vi "ui.vi"() -> ()   [LabVIEW 2018]
uses:
  control/clusterPlatformProfile.ctl
  control/clusterPlatformProfileTheta.ctl
  control/clusterPosition.ctl
  control/clusterPeriod.ctl
  control/clusterSensorState.ctl
  control/clusterPlatformState.ctl
  control/clusterTotalState.ctl
  control/enumTcpCommand.ctl
  <vilib>/Utility/miscctls.llb/LVRectTypeDef.ctl
  control/clusterCustomString.ctl
  <vilib>/Utility/miscctls.llb/LVBoundsTypeDef.ctl
  <vilib>/Utility/miscctls.llb/LVPositionTypeDef.ctl
  control/enumSensorType.ctl
  <vilib>/Utility/miscctls.llb/LVPointTypeDef.ctl
  control/enumFgvFunction.ctl
  <vilib>/Utility/sysdir.llb/System Directory Type.ctl
panel:
  out "Total State":T1={"Sensor State"={"Front"=0.0, "Rear"=0.0, "Right(F)"=0.0, "Righ(R)"=0.0}, "Position State"={"X"=1.0, "Y"=2.0, "Theta"=3.0}, "Platform State"={"Mode"=0, "State"=0}} {"Platform State"."Mode" format="%.0x"; "Platform State"."State" format="%.0x"}
  in  "sensor":T5
  in  "File Name":string
  in  "Save":bool
  in  "Init Platform":bool
  in  "AGV E-Stop":bool
  out "connect?":bool
  out "rx(ms)":u32
  out "tx(ms)":u32
  out "retry":i32
  in  "Tab Control":T6(tab)
  in  "AGV CCW":bool
  in  "AGV CW":bool
  in  "AGV Left":bool
  in  "ARV Right":bool
  in  "AGV Rear":bool
  in  "AGV Front":bool
  in  "Jog Control Velocity Profile Send":bool
  in  "Jog Control Velocity Profile":cluster{"X":T7, "Y":T7, "Theta":T8}={"X"={"Vel/s)"=0.05, "Acc(m/s^2)"=0.1, "Max Vel(m/s)"=0.5}, "Y"={"Vel/s)"=0.05, "Acc(m/s^2)"=0.1, "Max Vel(m/s)"=0.5}, "Theta"={"Vel(deg/s)"=1.0, "Acc(deg/s^2)"=1.0, "Max V(deg/s)"=30.0}}
  out "pos 4":T9(graph)
  out "vel 4":cluster{"value":dbl, "value":dbl, "value":dbl}(graph)
  in  "Position Control Veclocity Profile":cluster{"X":T7, "Y":T7, "Theta":T8}={"X"={"Vel/s)"=0.05, "Acc(m/s^2)"=0.1, "Max Vel(m/s)"=0.5}, "Y"={"Vel/s)"=0.02, "Acc(m/s^2)"=0.02, "Max Vel(m/s)"=0.5}, "Theta"={"Vel(deg/s)"=1.0, "Acc(deg/s^2)"=1.0, "Max V(deg/s)"=30.0}}
  out "vel 3":cluster{"value":dbl, "value":dbl, "value":dbl}(graph)
  in  "Position Control Veclocity Profile Send":bool
  in  "Position Send":bool
  in  "Position":T3
  in  "Pos Control Start":bool
  out "pos 3":T9(graph)
  in  "State Tab Control":enum32{"Request", "Monitor", "Whisper"}(tab)
  out "Get Total(Recv ms)":u32(graph)
  in  "Whisper Data":T10={"Period(ms)"=100}
  in  "Total Data":T10={"Period(ms)"=100}
  in  "Get Total State":bool
  out "Get Total(Recv ms)":u32(graph)
  in  "Get WhisperState":bool
  out "Whisper 1":T11[](array[typedef])
  out "Whisper 2":T11[](array[typedef])
  in  "RecipeLab Tab Control":enum32{"1", "2", "3", "4", "5"}(tab)
  in  "tx string":string
  in  "saving?":bool
  out "tx_packet":string
  out "rx_packet":string
  out "roscore(std out)":string
  out "roscore(std err)":string
  out "roscore(ret)":i32
  out "roscore(err)":errorcluster
  out "rqt(err)":errorcluster
  out "rqt(ret)":i32
  out "rqt(std err)":string
  out "rqt(std out)":string
  in  "roscore":bool
  in  "rqt":bool
  in  "address":string="127.0.0.1"
  in  "port":u16=10100
  in  "tcp rx close?":bool
  in  "send":bool
  out "tx_packet ts":timestamp format="%<%H:%M:%S%3u>T"
  out "rx_packet ts":timestamp format="%<%H:%M:%S%3u>T"
  out "STREAM":timestamp format="%<%H:%M:%S%3u>T"
  out "STREAM Command":T12
  out "ONE":timestamp format="%<%H:%M:%S%3u>T"
  out "ONE Command":T12
  out "RES ts":timestamp format="%<%H:%M:%S%3u>T"
  out "RES Command":T12
  out "ACK Command":T12
  out "ACK ts":timestamp format="%<%H:%M:%S%3u>T"
  in  "Maximize":bool
  out "stop":bool
  in  "AGV Stop(Jog)":bool caption="AGV Stop"
  in  "AGV Stop(Position Control)":bool caption="AGV Stop"
  in  "Command":T12=enum."Set Control Mode"
  in  "Set Control Mode":bool
  in  "Normal Stop(E-Stop)":bool
  in  "Set Jog Control Mode":bool
  in  "Set Position Control Mode":bool
  in  "Position Data":T10={"Period(ms)"=100}
  in  "Sensor Data":T10={"Period(ms)"=100}
  in  "Platform Data":T10={"Period(ms)"=100}
  out "Get Sensor(Recv ms)":u32(graph)
  out "Get Platform(Recv ms)":u32(graph)
  out "Get Position(Recv ms)":u32(graph)
  in  "Get Position State":bool
  in  "Get Sensor State":bool
  in  "Get Platform State":bool
  out "Sensor State":T2
  out "Platform State":T4
  out "Position State":T3={"X"=1.0, "Y"=2.0, "Theta"=3.0}
  in  "Front Panel Window Bounds":T13={"Left"=0, "Top"=27, "Right"=1024, "Bottom"=768}
  out "Position 2":T14
  out "Bounds":T15
  out "Array":cluster{"height":i16, "width":i16}[](array[cluster])
  out "Front Panel Window:Panel Bounds":T13
  out "Front Panel Window:Window Bounds":T13
  # "\"-- mode --\n0xA0: 조그(Jog)\n0xA1: 위치(Pos)\n0xAF: 초기화(Init)\n0xAE: 대기(Ready)\n-- state --\n0xB0: 대기(Ready)\n0xB1: 동작(Run)\""
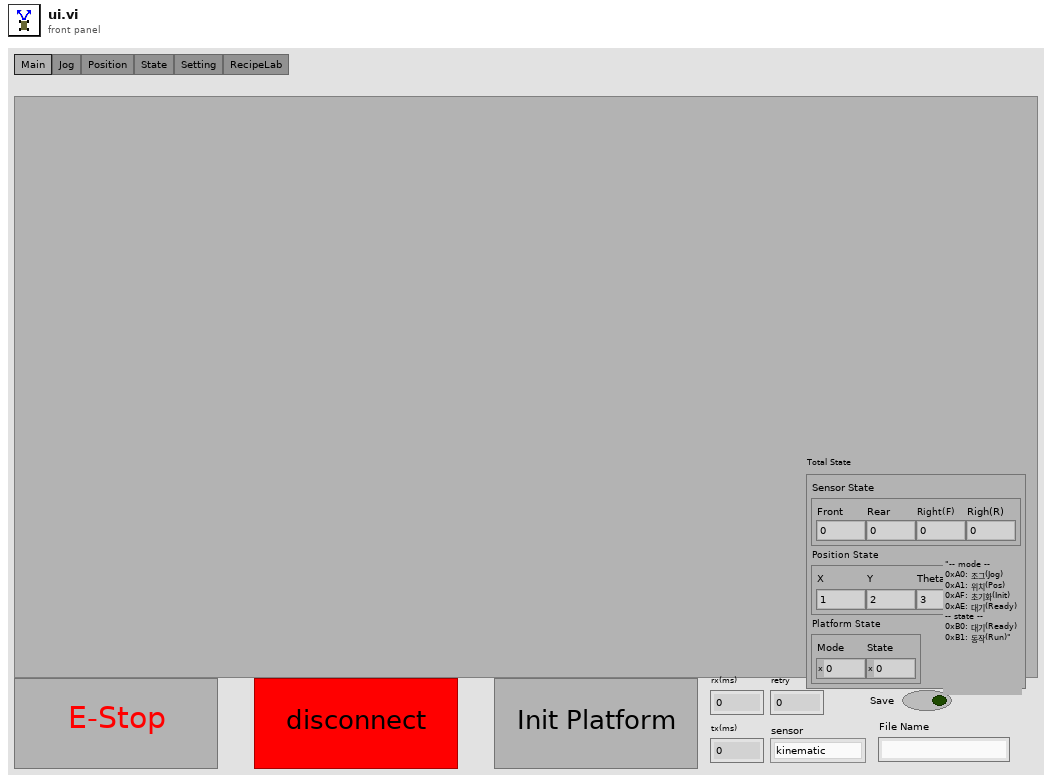
[diagram p1: front panel]
types:
  T1 = typedef "clusterTotalState.ctl" = cluster{"Sensor State":T2, "Position State":T3, "Platform State":T4}
  T2 = typedef "clusterSensorState.ctl" = cluster{"Front":dbl, "Rear":dbl, "Right(F)":dbl, "Righ(R)":dbl}
  T3 = typedef "clusterPosition.ctl" = cluster{"X":dbl, "Y":dbl, "Theta":dbl}
  T4 = typedef "clusterPlatformState.ctl" = cluster{"Mode":i32, "State":i32}
  T5 = typedef "enumSensorType.ctl" = enum16{"kinematic", "1d lidar", "fusion"}
  T6 = enum32{"Main", "Jog", "Position", "State", "Setting", "RecipeLab"}
  T7 = typedef "clusterPlatformProfile.ctl" = cluster{"Vel/s)":dbl, "Acc(m/s^2)":dbl, "Max Vel(m/s)":dbl}
  T8 = typedef "clusterPlatformProfileTheta.ctl" = cluster{"Vel(deg/s)":dbl, "Acc(deg/s^2)":dbl, "Max V(deg/s)":dbl}
  T9 = cluster{"value":dbl, "value":dbl, "value":dbl, "value":dbl, "value":dbl, "value":dbl}
  T10 = typedef "clusterPeriod.ctl" = cluster{"Period(ms)":i32}
  T11 = typedef "clusterCustomString.ctl" = cluster{"subject":string, "value":dbl}
  T12 = typedef "enumTcpCommand.ctl" = enum16{"None", "Stop", "E-Stop", "Set Position Control Mode", "Set Jog Control Mode", "Set Control Mode", "Set Jog Control Profile Parameter", "Set Position Control Profile Parameter", "Set Jog State", "Set Position", "Start Position Control", "Get Total State", "Get Platform State", "Get Sensor State", "Get Position State", "Init Platform", "Get Whisper State", "Set Sensor"}
  T13 = typedef "LVRectTypeDef.ctl" = cluster{"Left":i16, "Top":i16, "Right":i16, "Bottom":i16}
  T14 = typedef "LVPositionTypeDef.ctl" = cluster{"Left":i32, "Top":i32}
  T15 = typedef "LVBoundsTypeDef.ctl" = cluster{"Width":u32, "Height":u32}
  T16 = enum32{"invalid app kind", "Development System", "Run Time System", "Student Edition", "Embedded LabVIEW", "Evaluation", "Custom"}
  T17 = typedef "LVPointTypeDef.ctl" = cluster{"Horizontal":i16, "Vertical":i16}
  T18 = typedef "enumFgvFunction.ctl" = enum16{"Open", "Read", "Check", "Write", "Close"}
  T19 = cluster{"subject":u64, "subject":i64, "val_dbl":dbl}[]
  T20 = typedef "System Directory Type.ctl" = i32
  T21 = cluster{"[0]":u32, "[1]":u32, "[2]":u32, "[3]":u32, "[4]":u32, "[5]":u32}
  T22 = enum16{"Always On", "Always Off", "Off While Running"}
  T23 = enum16{"Standard", "Buffered", "CRLF", "Immediate"}
  T24 = cluster{cluster{dbl, dbl, dbl, dbl}, cluster{dbl, dbl, dbl}, cluster{i32, i32}}
  T25 = cluster{"double[0]":dbl, "double[1]":dbl, "double[2]":dbl, "double[3]":dbl}
  T26 = cluster{"double[0]":dbl, "double[1]":dbl, "double[2]":dbl}
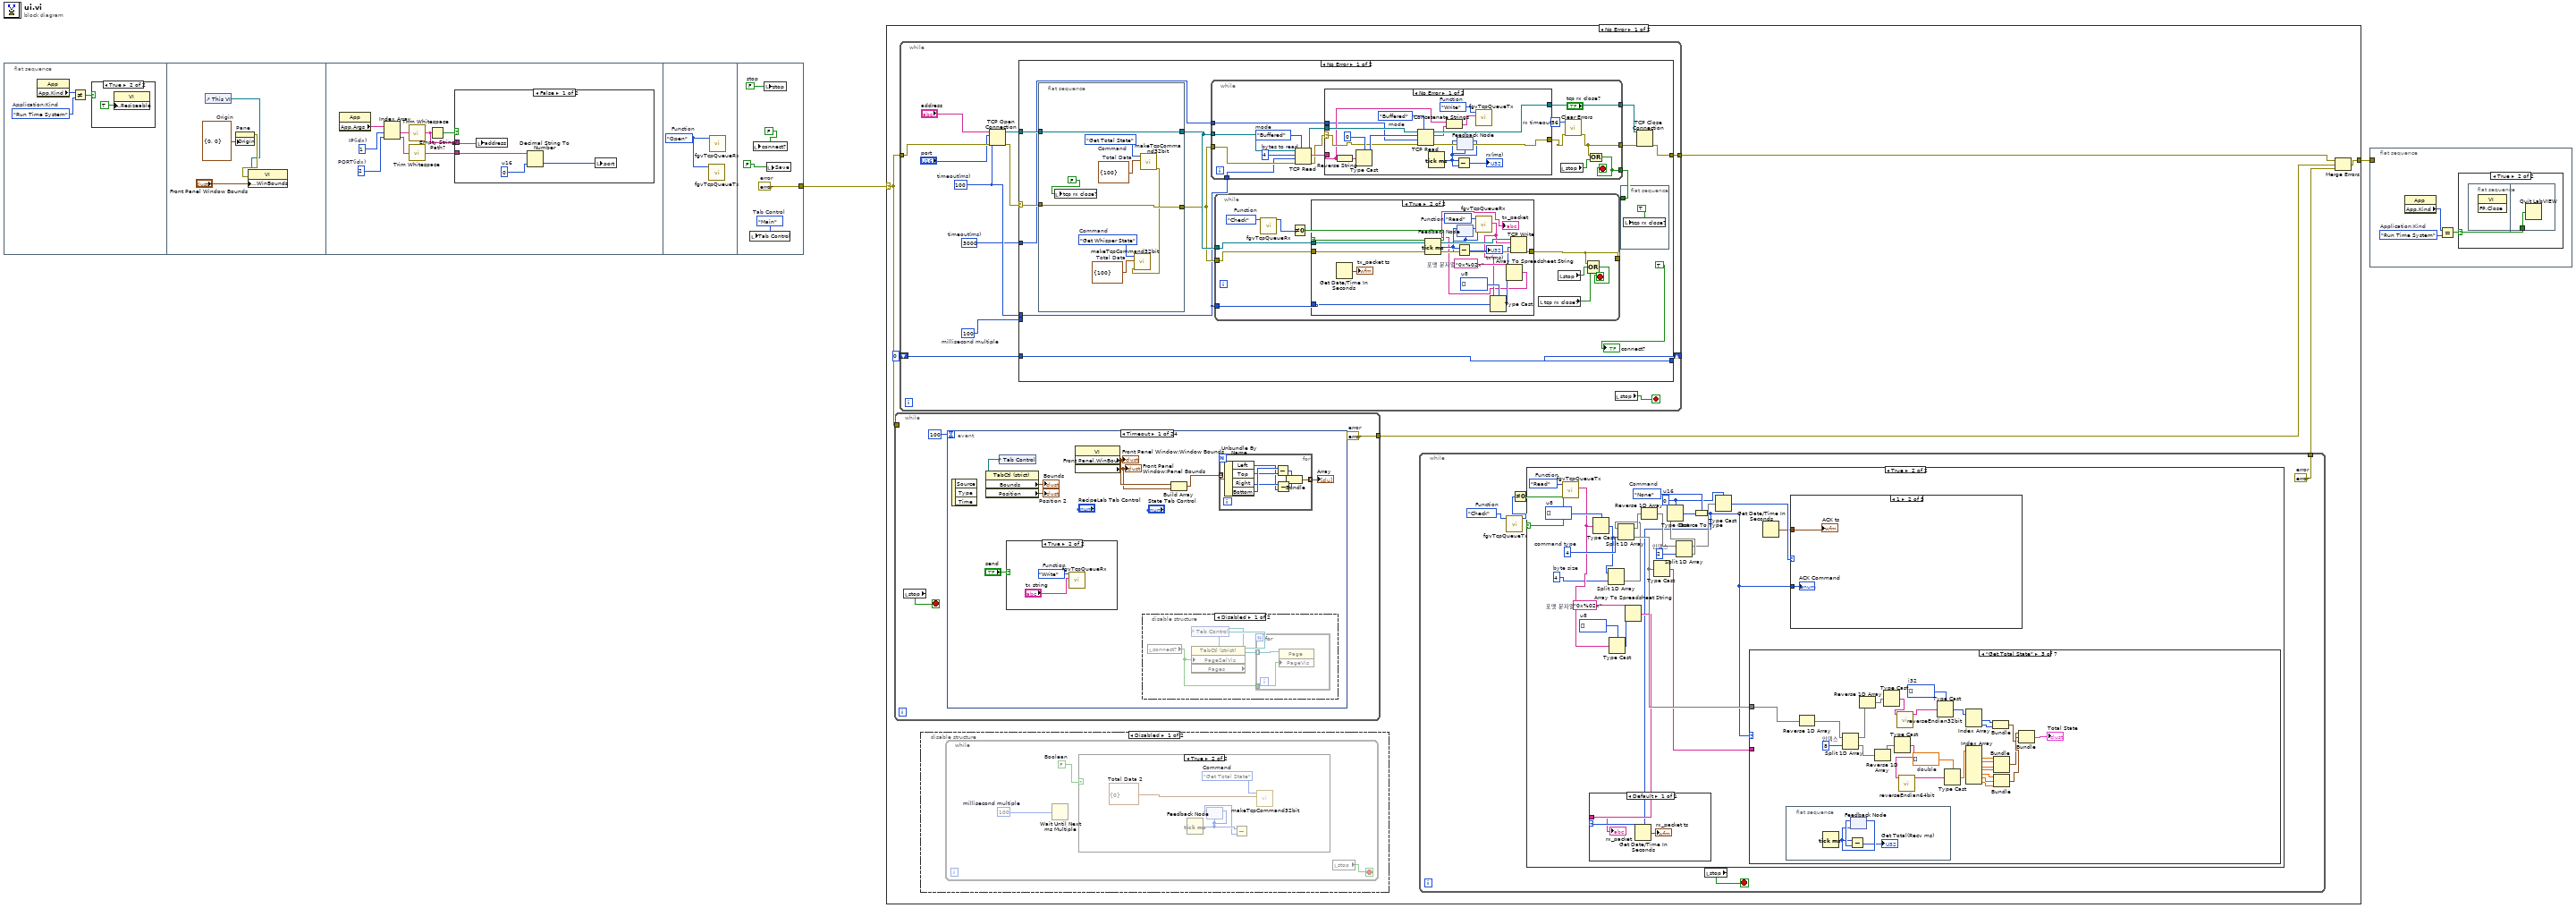
[diagram p0: block diagram]
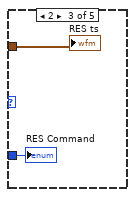
[diagram p6: hidden frame]
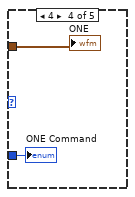
[diagram p7: hidden frame]
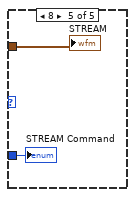
[diagram p8: hidden frame]
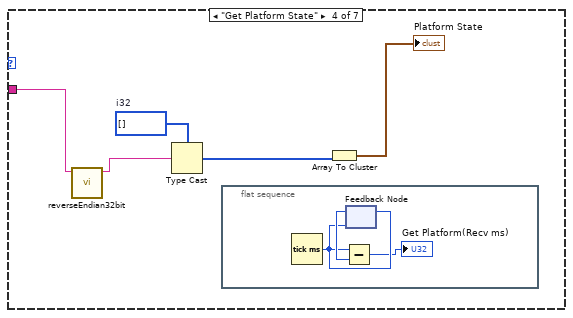
[diagram p11: hidden frame]
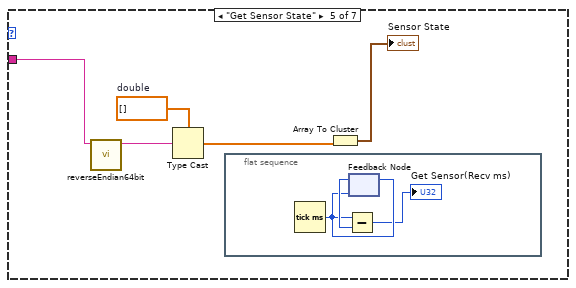
[diagram p12: hidden frame]
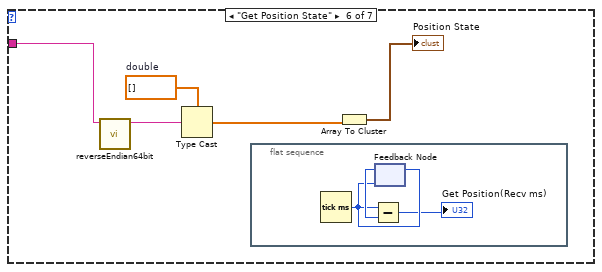
[diagram p13: hidden frame]
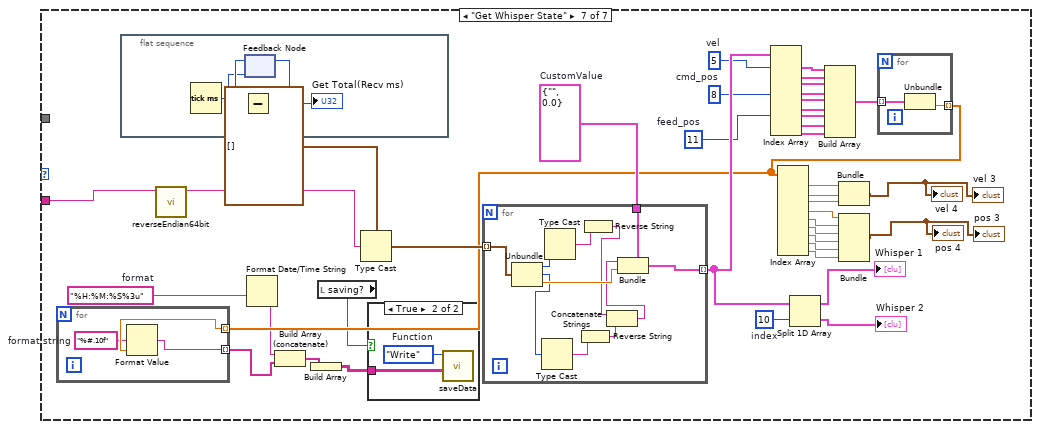
[diagram p14: hidden frame]
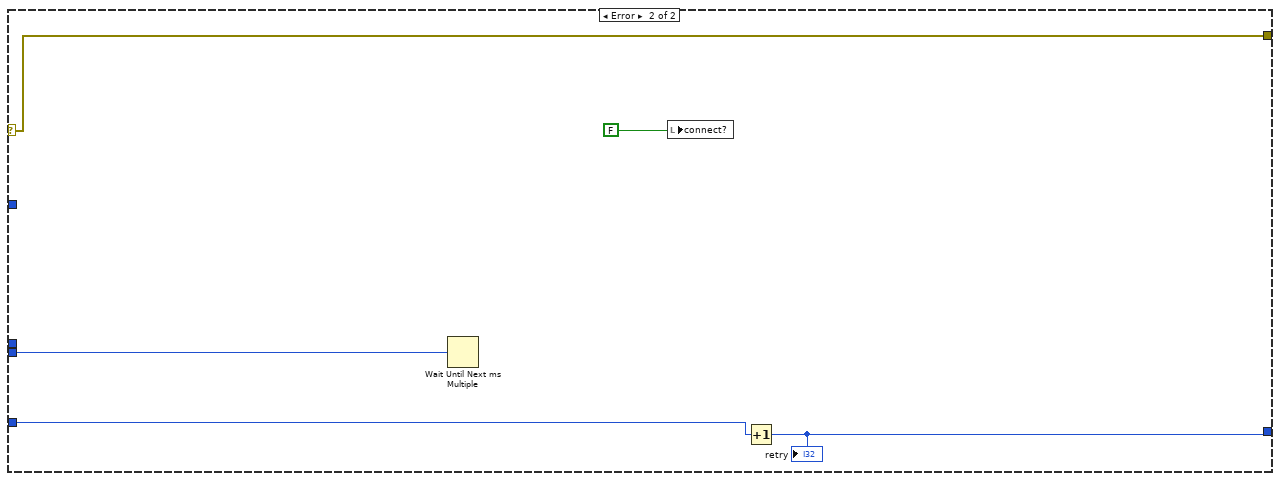
[diagram p18: hidden frame]
diagram:
  n1 = flat-sequence {
    tunnel: [w27] -> w1
    frame #0 {
      w3 = T16."Run Time System"  # Application:Kind
      n2 = property class="App"() -> ("App.Kind"=w4:T16)  [unwired: 2 in, 2 out]
      n3 = Not Equal?(x=w4, y=w3) -> (x != y?=w5:bool)
      n4 = case shown="True" w5 {
        frame False {
        }
        frame True {
          n5 = property class="VI"("Front Panel.Resizeable"=TRUE) -> ()  [unwired: 2 in, 2 out]
        }
      }
    }
    frame #1 {
      w10 = T17 {"Horizontal"=0, "Vertical"=0}  # Origin
      n6 = control-ref of="This VI"() -> (w8:refnum<vi>)
      n7 = property on="Pane" class="Pane"("Origin"=w10) -> (error out=w9:errorcluster)  [unwired: 2 in, 1 out]
      n8 = property on="Property Node" class="VI"(reference=w8, error in=w9, "Front Panel.WinBounds"="Front Panel Window Bounds") -> ()  [unwired: 2 out]
    }
    frame #2 {
      w16 = 2  # PORT(idx)
      w17 = 1  # IP(idx)
      n9 = property class="App"() -> ("App.Args"=w18:string[])  [unwired: 2 in, 2 out]
      n10 = Index Array(array=w18, index #1=w17, index #2=w16) -> (element #1=w15:string, element #2=w14:string)
      n11 = call <vilib>:"Trim Whitespace.vi"("string"=w15) -> ("trimmed string"=w13:string)  [unwired: 1 in]
      n12 = call <vilib>:"Trim Whitespace.vi"("string"=w14) -> ("trimmed string"=w12:string)  [unwired: 1 in]
      n13 = Empty String/Path?(string/path=w13) -> (empty?=w11:bool)
      n14 = case shown="False" w11 {
        tunnel: w13 -> [w22 _]
        tunnel: w12 -> [w21 _]
        frame False {
          w19 = u16 0  # u16
          n15 = local write "address"(w22) -> ()
          n16 = Decimal String To Number(string=w21, default (0L)=w19) -> (number=w20:u16)  [unwired: 1 in, 1 out]
          n17 = local write "port"(w20) -> ()
        }
        frame True {
        }
      }
    }
    frame #3 {
      w23 = enumFgvFunction."Open"  # Function
      n18 = call "fgvTcpQueueTx.vi"("Function"=w23) -> ()  [unwired: 8 in, 3 out]
      n19 = call "fgvTcpQueueRx.vi"("Function"=w23) -> ()  [unwired: 8 in, 3 out]
    }
    frame #4 {
      w24 = T6."Main"  # Tab Control
      w27 = errorcluster {"status"=FALSE, "code"=0, "source"=""}  # error
      w28 = FALSE  # stop
      n20 = local write "Tab Control"(w24) -> ()
      n21 = local write "connect?"(FALSE) -> ()
      n22 = local write "stop"(w28) -> ()
      n23 = local write "Save"(FALSE) -> ()
    }
  }
  n24 = case shown="No Error" w1 {
    selector: w1 -> [w32 w422]
    tunnel: [w33 w422] -> w2
    frame No Error {
      n25 = while {
        tunnel: w32 -> [_]
        tunnel: [w293] -> w34
        stop <- w295 stop-if-true
        w293 = errorcluster {"status"=FALSE, "code"=0, "source"=""}  # error
        n26 = local read "stop"() -> (w295:bool)
        n27 = event shown="[0] Timeout" {
          selector: _ -> [_ _ _ _ _ _ _ _ _ _ _ _ _ _ _ _ _ _ _ _ _ _ _ _]
          dyn-events: _ -> [_ _ _ _ _ _ _ _ _ _ _ _ _ _ _ _ _ _ _ _ _ _ _ _]
          timeout: 100 -> [_ _ _ _ _ _ _ _ _ _ _ _ _ _ _ _ _ _ _ _ _ _ _ _]
          event Timeout {
            n28 = event-data() -> ()  [unwired: 1 in, 3 out]
            n29 = control-ref of="Tab Control"() -> (w299:refnum<vi>)
            n30 = property on="Property Node" class="TabCtl (strict)"(reference=w299) -> ("Bounds"=→"Bounds":T15, "Position"=→"Position 2":T14)  [unwired: 1 in, 2 out]
            n31 = case shown="True" "send" {
              frame False {
              }
              frame True {
                w305 = enumFgvFunction."Write"  # Function
                n32 = call "fgvTcpQueueRx.vi"("Write"="tx string", "Function"=w305) -> ()  [unwired: 7 in, 3 out]
              }
            }
            n33 = property on="Property Node" class="VI"() -> ("Front Panel.WinBounds"=w303:T13, "Front Panel.PanelBounds"=w302:T13)  [unwired: 2 in, 2 out]
            "Front Panel Window:Window Bounds" <- w303
            "Front Panel Window:Panel Bounds" <- w302
            n34 = disable-structure shown="Disabled" {
              frame Disabled {
                n35 = local read "connect?"() -> (w306:bool)
                n36 = control-ref of="Tab Control"() -> (w308:refnum<vi>)
                n37 = property class="TabCtl (strict)"(reference=w308, "PageSelVis"=w306) -> ("Pages"=w307:refnum<vi>[])  [unwired: 1 in, 2 out]
                n38 = for {
                  tunnel: w307 -> [w310] mode=indexing
                  tunnel: w306 -> [w309]
                  n39 = property class="Page"(reference=w310, "PageVis"=w309) -> ()  [unwired: 1 in, 2 out]
                }
              }
              frame Enabled {
              }
            }
            n40 = Build Array(w303, w302) -> (w301:T13[])
            n41 = for {
              tunnel: w301 -> [w318] mode=indexing
              tunnel: [w311] -> w300 mode=indexing
              n42 = Unbundle By Name(w318) -> ("Left"=w314:i16, "Top"=w316:i16, "Right"=w315:i16, "Bottom"=w317:i16)
              n43 = Subtract(x=w317, y=w316) -> (x-y=w313:i16)
              n44 = Subtract(x=w315, y=w314) -> (x-y=w312:i16)
              n45 = Bundle(w313, w312) -> (w311:cluster{i16, i16})  [unwired: 1 in]
            }
            "Array" <- w300
          }
          event Value Change {
            w321 = enumTcpCommand."Set Sensor"  # Command
            n46 = event-data() -> ()  [unwired: 1 in, 6 out]
            n47 = To Unsigned Long Integer(number="sensor") -> (unsigned 32bit integer=w319:u32)
            n48 = call "makeTcpCommand32bit.vi"("Variant"=w319, "Command"=w321) -> ()  [unwired: 7 in, 3 out]
          }
          event "Tab Control": Value Change {
            n49 = event-data() -> ("OldVal"=w324:T6, "NewVal"=w322:T6)  [unwired: 1 in, 4 out]
            n50 = Not Equal?(x=w324, y=w322) -> (x != y?=w323:bool)
            n51 = case shown="True" w323 {
              tunnel: w322 -> [_ w325]
              frame False {
              }
              frame True {
                n52 = case shown="\"Jog\"" w325 {
                  frame Default {
                  }
                  frame "Jog" {
                    w327 = enumTcpCommand."Set Jog Control Profile Parameter"  # Command
                    w329 = enumTcpCommand."Set Jog Control Mode"  # Command
                    n53 = call "makeTcpCommand32bit.vi"("Command"=w329) -> ("error out"=w326:errorcluster)  [unwired: 8 in, 2 out]
                    n54 = local read "Jog Control Velocity Profile"() -> (w328:cluster{"X":T7, "Y":T7, "Theta":T8})
                    n55 = call "makeTcpCommand64bit.vi"("error in"=w326, "Variant"=w328, "Command"=w327) -> ()  [unwired: 6 in, 3 out]
                  }
                  frame "Position" {
                    w331 = enumTcpCommand."Set Position Control Profile Parameter"  # Command
                    w333 = enumTcpCommand."Set Position Control Mode"  # Command
                    n56 = call "makeTcpCommand32bit.vi"("Command"=w333) -> ("error out"=w330:errorcluster)  [unwired: 8 in, 2 out]
                    n57 = local read "Position Control Veclocity Profile"() -> (w332:cluster{"X":T7, "Y":T7, "Theta":T8})
                    n58 = call "makeTcpCommand64bit.vi"("error in"=w330, "Variant"=w332, "Command"=w331) -> ()  [unwired: 6 in, 3 out]
                  }
                }
              }
            }
          }
          event "Save": Value Change {
            n59 = event-data() -> ("NewVal"=w335:bool)  [unwired: 1 in, 5 out]
            n60 = case shown="False" w335 {
              tunnel: [FALSE TRUE] -> w334
              frame False {
                w337 = enumFgvFunction."Close"  # Function
                n61 = call "saveData.vi"("Function"=w337) -> ()  [unwired: 8 in, 3 out]
              }
              frame True {
                w338 = "_"  # string
                w343 = string[][] [["timestamp", "vel.x", "vel.y", "vel.rx", "cmdx", "cmdy", "cmdz", "feedx", "feedy", "feedz"]]  # header
                w346 = T20 0 items=["User Home"=0, "User Desktop"=1, "User Documents"=2, "User Application Data"=3, "User Preferences"=4, "User Temporary"=5, "Public Documents"=6, "Public Application Data"=7, "Public Preferences"=8, "Public Cache"=13, "System Core Libraries"=9, "System Installed Libraries"=10, "Application Files"=11, "Boot Volume Root"=12]  # system directory type
                w348 = enumFgvFunction."Open"  # Function
                n62 = call <vilib>:"Get System Directory.vi"("system directory type"=w346) -> ("system directory"=w345:path)  [unwired: 10 in]
                n63 = control-ref of="This VI"() -> (w342:refnum<vi>)
                n64 = Format Date/Time String(time format string (%c)="%Y%m%d_%H%M%S") -> (date/time string=w341:string)  [unwired: 2 in]
                n65 = Concatenate Strings(w341, w338, "File Name") -> (w339:string)
                n66 = call "saveData.vi"("file name"=w339, "이미지 저장 VI"=w342, "file path 경로"=w345, "header"=w343, "Function"=w348) -> ()  [unwired: 4 in, 3 out]
              }
            }
            n67 = local write "saving?"(w334) -> ()
          }
          event "roscore": Value Change {
            n68 = event-data() -> ()  [unwired: 1 in, 6 out]
            n69 = call <vilib>:"System Exec.vi"("wait until completion? (T)"=FALSE, "command line"="roscore") -> ("error out"=→"roscore(err)":errorcluster, "return code"=→"roscore(ret)":i32, "standard error"=→"roscore(std err)":string, "standard output"=→"roscore(std out)":string)  [unwired: 6 in]
          }
          event "Position Control Veclocity Profile Send": Value Change {
            w356 = enumTcpCommand."Set Position Control Profile Parameter"  # Command
            n70 = event-data() -> ()  [unwired: 1 in, 6 out]
            n71 = call "makeTcpCommand64bit.vi"("Variant"="Position Control Veclocity Profile", "Command"=w356) -> ()  [unwired: 7 in, 3 out]
          }
          event "Jog Control Velocity Profile Send": Value Change {
            w358 = enumTcpCommand."Set Jog Control Profile Parameter"  # Command
            n72 = event-data() -> ()  [unwired: 1 in, 6 out]
            n73 = call "makeTcpCommand64bit.vi"("Variant"="Jog Control Velocity Profile", "Command"=w358) -> ()  [unwired: 7 in, 3 out]
          }
          event "AGV Front", "AGV Rear", "ARV Right", "AGV Left", "AGV CW", "AGV CCW": Value Change {
            w364 = enumTcpCommand."Set Jog State"  # Command
            n74 = event-data() -> ()  [unwired: 1 in, 6 out]
            n75 = Build Array("AGV Front", "AGV Rear", "AGV Left", "ARV Right", "AGV CW", "AGV CCW") -> (w365:bool[])
            n76 = Boolean To (0,1)(Boolean=w365) -> (0, 1=w363:i16[])
            n77 = To Unsigned Long Integer(number=w363) -> (unsigned 32bit integer=w360:u32[])
            n78 = Array To Cluster(array=w360) -> (cluster=w359:T21)
            n79 = call "makeTcpCommand32bit.vi"("Variant"=w359, "Command"=w364) -> ()  [unwired: 7 in, 3 out]
          }
          event "Set Jog Control Mode": Value Change {
            w370 = enumTcpCommand."Set Jog Control Mode"  # Command
            n80 = event-data() -> ()  [unwired: 1 in, 6 out]
            n81 = call "makeTcpCommand32bit.vi"("Command"=w370) -> ()  [unwired: 8 in, 3 out]
          }
          event "Set Control Mode": Value Change {
            w374 = enumTcpCommand."Set Control Mode"  # Command
            n82 = event-data() -> ()  [unwired: 1 in, 6 out]
            n83 = To Unsigned Long Integer(number="Command") -> (unsigned 32bit integer=w372:u32)
            n84 = Bundle(w372) -> (w371:cluster{u32})  [unwired: 1 in]
            n85 = call "makeTcpCommand32bit.vi"("Variant"=w371, "Command"=w374) -> ()  [unwired: 7 in, 3 out]
          }
          event "Init Platform": Value Change {
            w375 = enumTcpCommand."Init Platform"  # Command
            n86 = event-data() -> ()  [unwired: 1 in, 6 out]
            n87 = call "makeTcpCommand32bit.vi"("Command"=w375) -> ()  [unwired: 8 in, 3 out]
          }
          event "Set Position Control Mode": Value Change {
            w376 = enumTcpCommand."Set Position Control Mode"  # Command
            n88 = event-data() -> ()  [unwired: 1 in, 6 out]
            n89 = call "makeTcpCommand32bit.vi"("Command"=w376) -> ()  [unwired: 8 in, 3 out]
          }
          event "AGV E-Stop": Value Change {
            w377 = enumTcpCommand."E-Stop"  # Command
            n90 = event-data() -> ()  [unwired: 1 in, 6 out]
            n91 = call "makeTcpCommand32bit.vi"("Command"=w377) -> ()  [unwired: 8 in, 3 out]
          }
          event "Pos Control Start": Value Change {
            w378 = enumTcpCommand."Start Position Control"  # Command
            n92 = event-data() -> ()  [unwired: 1 in, 6 out]
            n93 = call "makeTcpCommand32bit.vi"("Command"=w378) -> ()  [unwired: 8 in, 3 out]
          }
          event "Get Total State": Value Change {
            w380 = enumTcpCommand."Get Total State"  # Command
            n94 = event-data() -> ()  [unwired: 1 in, 6 out]
            n95 = call "makeTcpCommand32bit.vi"("Variant"="Total Data", "Command"=w380) -> ()  [unwired: 7 in, 3 out]
          }
          event "Get Sensor State": Value Change {
            w382 = enumTcpCommand."Get Sensor State"  # Command
            n96 = event-data() -> ()  [unwired: 1 in, 6 out]
            n97 = call "makeTcpCommand32bit.vi"("Variant"="Sensor Data", "Command"=w382) -> ()  [unwired: 7 in, 3 out]
          }
          event "Get Position State": Value Change {
            w384 = enumTcpCommand."Get Position State"  # Command
            n98 = event-data() -> ()  [unwired: 1 in, 6 out]
            n99 = call "makeTcpCommand32bit.vi"("Variant"="Position Data", "Command"=w384) -> ()  [unwired: 7 in, 3 out]
          }
          event "Get Platform State": Value Change {
            w386 = enumTcpCommand."Get Platform State"  # Command
            n100 = event-data() -> ()  [unwired: 1 in, 6 out]
            n101 = call "makeTcpCommand32bit.vi"("Variant"="Platform Data", "Command"=w386) -> ()  [unwired: 7 in, 3 out]
          }
          event "Get WhisperState": Value Change {
            w388 = enumTcpCommand."Get Whisper State"  # Command
            n102 = event-data() -> ()  [unwired: 1 in, 6 out]
            n103 = call "makeTcpCommand32bit.vi"("Variant"="Whisper Data", "Command"=w388) -> ()  [unwired: 7 in, 3 out]
          }
          event "AGV Stop(Jog)", "AGV Stop(Position Control)": Value Change {
            n104 = event-data() -> ("CtlRef"=w391:refnum<vi>, "NewVal"=w389:bool)  [unwired: 1 in, 4 out]
            n105 = property class="Bool (strict)"(reference=w391) -> ("Label.Text"=w390:string)  [unwired: 1 in, 2 out]
            n106 = case shown="\"AGV Stop(Position Control)\"" w390 {
              tunnel: w389 -> [_ w396 w397]
              frame Default {
              }
              frame "AGV Stop(Jog)" {
                n107 = local write "AGV Stop(Position Control)"(w396) -> ()
              }
              frame "AGV Stop(Position Control)" {
                n108 = local write "AGV Stop(Jog)"(w397) -> ()
              }
            }
            n109 = case shown="True" w389 {
              frame False {
              }
              frame True {
                w394 = enumTcpCommand."Stop"  # Command
                n110 = Boolean To (0,1)(Boolean="Normal Stop(E-Stop)") -> (0, 1=w395:i16)
                n111 = To Unsigned Long Integer(number=w395) -> (unsigned 32bit integer=w393:u32)
                n112 = call "makeTcpCommand32bit.vi"("Variant"=w393, "Command"=w394) -> ()  [unwired: 7 in, 3 out]
              }
            }
          }
          event "Maximize": Value Change {
            w398 = T22."Off While Running"  # Horizontal Scrollbar Visibility
            w401 = FALSE  # Tool Bar:Visible
            w402 = FALSE  # Front Panel Window:Show Menu Bar
            w403 = T13 {"Left"=0, "Top"=27, "Right"=1024, "Bottom"=768}  # Front Panel Window:Panel Bounds
            w404 = TRUE  # Front Panel Window:Is Frontmost
            n113 = event-data() -> ()  [unwired: 1 in, 6 out]
            n114 = control-ref of="This VI"() -> (w405:refnum<vi>)
            n115 = property class="VI" props=["Front Panel.IsFrontmost", "Front Panel.PanelBounds", "Front Panel.ShowMenuBar", "TB.Visible", "Clone Name"](reference=w405, "Front Panel.IsFrontmost"=w404, "Front Panel.PanelBounds"=w403, "Front Panel.ShowMenuBar"=w402, "TB.Visible"=w401) -> (error out=w400:errorcluster)  [unwired: 1 in, 2 out]
            n116 = control-ref of="Pane"() -> (w399:refnum<vi>)
            n117 = property class="Pane"(reference=w399, error in=w400, "HorizScrollbarVisibility"=w398, "VertScrollbarVisibility"=w398) -> ()  [unwired: 2 out]
          }
          event "Position Send": Value Change {
            w407 = enumTcpCommand."Set Position"  # Command
            n118 = event-data() -> ()  [unwired: 1 in, 6 out]
            n119 = call "makeTcpCommand64bit.vi"("Variant"="Position", "Command"=w407) -> ()  [unwired: 7 in, 3 out]
          }
          event "rqt": Value Change {
            n120 = event-data() -> ()  [unwired: 1 in, 6 out]
            n121 = call <vilib>:"System Exec.vi"("wait until completion? (T)"=FALSE, "command line"="rqt") -> ("error out"=→"rqt(err)":errorcluster, "return code"=→"rqt(ret)":i32, "standard error"=→"rqt(std err)":string, "standard output"=→"rqt(std out)":string)  [unwired: 6 in]
          }
          event Panel Close? {
            w414 = TRUE  # stop
            n122 = event-data() -> ()  [unwired: 1 in, 4 out]
            n123 = disable-structure shown="Enabled" {
              disable-tunnel: [w416 TRUE] -> w415
              frame Disabled {
                w418 = T16."Run Time System"  # Application:Kind
                n124 = property class="App"() -> ("App.Kind"=w419:T16)  [unwired: 2 in, 2 out]
                n125 = Equal?(x=w419, y=w418) -> (x = y?=w417:bool)
                n126 = Not(x=w417) -> (.not. x?=w416:bool)
              }
              frame Enabled {
              }
            }
            n127 = event-data("Discard?"=w415) -> ()  [unwired: 1 in, 1 out]
            "stop" <- w414
          }
        }
      }
      n128 = while {
        tunnel: w32 -> [w207]
        tunnel: [w206] -> w31
        shift-right: [w201] -> _
        shift-left: 0 -> [w200]
        stop <- w208 stop-if-true
        w197 = 3000  # timeout(ms)
        w199 = u32 100  # millisecond multiple
        w198 = 100  # timeout(ms)
        n129 = TCP Open Connection(address="address", remote port or service name="port", timeout ms (60000)=w198, error in (no error)=w207) -> (connection ID=w203:refnum<k5>, error out=w202:errorcluster)  [unwired: 1 in]
        n130 = case shown="No Error" w202 {
          selector: w202 -> [w212 w292]
          tunnel: [w219 w292] -> w206
          tunnel: w203 -> [w214 _]
          tunnel: [w217 w290] -> w201
          tunnel: w200 -> [w217 w291]
          tunnel: w199 -> [_ w288]
          tunnel: w198 -> [w211 _]
          tunnel: w197 -> [w210 _]
          frame No Error {
            n131 = flat-sequence {
              tunnel: [w229] -> w215
              tunnel: w214 -> [w229]
              tunnel: [w228] -> w213
              tunnel: w212 -> [w228]
              frame #0 {
                w225 = T10 {"Period(ms)"=100}  # Total Data
                w224 = enumTcpCommand."Get Whisper State"  # Command
                w226 = T10 {"Period(ms)"=100}  # Total Data
                w227 = enumTcpCommand."Get Total State"  # Command
                n132 = local write "tcp rx close?"(FALSE) -> ()
                n133 = call "makeTcpCommand32bit.vi"("Variant"=w226, "Command"=w227) -> ("error out"=w223:errorcluster)  [unwired: 7 in, 2 out]
                n134 = call "makeTcpCommand32bit.vi"("error in"=w223, "Variant"=w225, "Command"=w224) -> ()  [unwired: 6 in, 3 out]
              }
            }
            n135 = while {
              tunnel: w213 -> [w269]
              tunnel: [w259] -> w220
              tunnel: w215 -> [w268]
              tunnel: [w262] -> w218
              tunnel: w211 -> [w257]
              tunnel: w210 -> [w256]
              tunnel: [w255] -> w209
              stop <- w255 stop-if-true
              w258 = 56  # rx timeout
              w266 = 4  # bytes to read
              w267 = T23."Buffered"  # mode
              n136 = TCP Read(connection ID=w268, bytes to read=w266, error in (no error)=w269, 7:w267, 9:w257) -> (connection ID out=w264:refnum<k5>, data out=w263:string, error out=w261:errorcluster)
              n137 = case shown="No Error" w261 {
                selector: w261 -> [w277 w287]
                tunnel: w264 -> [w284 w286]
                tunnel: w263 -> [w273 _]
                tunnel: [w280 w286] -> w262
                tunnel: [w279 w287] -> w260
                tunnel: w256 -> [w270 _]
                frame No Error {
                  w278 = enumFgvFunction."Write"  # Function
                  w285 = T23."Buffered"  # mode
                  n138 = Reverse String(1:w273) -> (0:w283:string)
                  n139 = Type Cast(type=0, x=w283) -> (*(type *) &x=w282:i32)
                  n140 = TCP Read(connection ID=w284, bytes to read=w282, error in (no error)=w277, 7:w285, 9:w270) -> (connection ID out=w280:refnum<k5>, data out=w272:string, error out=w279:errorcluster)
                  n141 = Tick Count (ms)() -> (millisecond timer value=w275:u32)
                  n142 = Concatenate Strings(w273, w272) -> (w271:string)
                  n143 = feedback #1(w275) -> (w274:u32)
                  n144 = Subtract(x=w275, y=w274) -> (x-y=→"rx(ms)":u32)
                  n145 = feedback-in #1(w275) -> ()
                  n146 = call "fgvTcpQueueTx.vi"("Write"=w271, "Function"=w278) -> ()  [unwired: 7 in, 3 out]
                }
                frame Error {
                }
              }
              n147 = local read "stop"() -> (w265:bool)
              n148 = call <vilib>:"Clear Errors.vi"("error in (no error)"=w260, "specific error code to clear (0: all)"=w258) -> ("error out"=w259:errorcluster)  [unwired: 4 in, 1 out]
              n149 = Compound Arithmetic op=OR(w259, w265) -> (w255:bool)
            }
            n150 = while {
              tunnel: w213 -> [w231]
              tunnel: [w239] -> _
              tunnel: w215 -> [w233]
              tunnel: w211 -> [w232]
              stop <- w237 stop-if-true
              w236 = enumFgvFunction."Check"  # Function
              n151 = call "fgvTcpQueueRx.vi"("Function"=w236) -> ("Count"=w235:i32)  [unwired: 8 in, 2 out]
              n152 = Not Equal To 0?(x=w235) -> (x != 0?=w234:bool)
              n153 = case shown="True" w234 {
                tunnel: [w240 w254] -> w239
                tunnel: w231 -> [w240 w253]
                tunnel: w233 -> [_ w252]
                tunnel: w232 -> [_ w242]
                frame False {
                }
                frame True {
                  w247 = "0x%02x"  # 포맷 문자열
                  w245 = u8[] []  # u8
                  w251 = enumFgvFunction."Read"  # Function
                  n154 = Get Date/Time In Seconds() -> (seconds since 1Jan1904=→"tx_packet ts":timestamp)
                  n155 = Tick Count (ms)() -> (millisecond timer value=w249:u32)
                  n156 = feedback #2(w249) -> (w248:u32)
                  n157 = Subtract(x=w249, y=w248) -> (x-y=→"tx(ms)":u32)
                  n158 = feedback-in #2(w249) -> ()
                  n159 = call "fgvTcpQueueRx.vi"("Function"=w251) -> ("Read"=w244:string)  [unwired: 8 in, 2 out]
                  n160 = Type Cast(type=w245, x=w244) -> (*(type *) &x=w246:u8[])
                  n161 = Array To Spreadsheet String(array=w246, 3:w247) -> (spreadsheet string=→"tx_packet":string)  [unwired: 1 in]
                  n162 = TCP Write(connection ID=w252, data in=w244, error in (no error)=w253, 9:w242) -> (error out=w254:errorcluster)  [unwired: 2 out]
                }
              }
              n163 = local read "tcp rx close?"() -> (w230:bool)
              n164 = local read "stop"() -> (w238:bool)
              n165 = Compound Arithmetic op=OR(w239, w238, w230) -> (w237:bool)
            }
            n166 = flat-sequence {
              tunnel: w209 -> [_]
              frame #0 {
                n167 = local write "tcp rx close?"(TRUE) -> ()
              }
            }
            n168 = TCP Close Connection(connection ID=w218, error in (no error)=w220) -> (error out=w219:errorcluster)  [unwired: 1 in, 1 out]
            "connect?" <- TRUE
          }
          frame Error {
            n169 = Wait Until Next ms Multiple(millisecond multiple=w288) -> ()  [unwired: 1 out]
            n170 = local write "connect?"(FALSE) -> ()
            n171 = Increment(x=w291) -> (x+1=w290:i32)
            "retry" <- w290
          }
        }
        n172 = local read "stop"() -> (w208:bool)
      }
      n173 = disable-structure shown="Disabled" {
        frame Disabled {
          n174 = while {
            stop <- w36 stop-if-true
            w35 = FALSE  # Boolean
            w37 = u32 100  # millisecond multiple
            n175 = Wait Until Next ms Multiple(millisecond multiple=w37) -> ()  [unwired: 1 out]
            n176 = case shown="True" w35 {
              frame False {
              }
              frame True {
                w41 = T10 {"Period(ms)"=0}  # Total Data 2
                w40 = enumTcpCommand."Get Total State"  # Command
                n177 = Tick Count (ms)() -> (millisecond timer value=w39:u32)
                n178 = feedback-in #3(w39) -> ()
                n179 = feedback #3(w39) -> (w38:u32)
                n180 = Subtract(x=w39, y=w38) -> ()  [unwired: 1 out]
                n181 = call "makeTcpCommand32bit.vi"("Variant"=w41, "Command"=w40) -> ()  [unwired: 7 in, 3 out]
              }
            }
            n182 = local read "stop"() -> (w36:bool)
          }
        }
        frame Enabled {
        }
      }
      n183 = while {
        tunnel: [w42] -> w29
        stop <- w45 stop-if-true
        w42 = errorcluster {"status"=FALSE, "code"=0, "source"=""}  # error
        w46 = enumFgvFunction."Check"  # Function
        n184 = call "fgvTcpQueueTx.vi"("Function"=w46) -> ("Count"=w44:i32)  [unwired: 8 in, 2 out]
        n185 = Not Equal To 0?(x=w44) -> (x != 0?=w43:bool)
        n186 = case shown="True" w43 {
          frame False {
          }
          frame True {
            w53 = 2  # 인덱스
            w55 = 4  # byte size
            w60 = "0x%02x"  # 포맷 문자열
            w62 = u8[] []  # u8
            w50 = u16 0  # u16
            w66 = enumTcpCommand."None"  # Command
            w68 = 4  # command type
            w69 = u8[] []  # u8
            w70 = enumFgvFunction."Read"  # Function
            n187 = call "fgvTcpQueueTx.vi"("Function"=w70) -> ("Read"=w58:string)  [unwired: 8 in, 2 out]
            n188 = Type Cast(type=w69, x=w58) -> (*(type *) &x=w57:u8[])
            n189 = Split 1D Array(array=w57, index=w55) -> (second subarray=w56:u8[])  [unwired: 1 out]
            n190 = Type Cast(type=w62, x=w58) -> (*(type *) &x=w61:u8[])
            n191 = Split 1D Array(array=w56, index=w68) -> (first subarray=w67:u8[], second subarray=w64:u8[])
            n192 = Array To Spreadsheet String(array=w61, 3:w60) -> (spreadsheet string=w59:string)  [unwired: 1 in]
            n193 = Reverse 1D Array(array=w67) -> (reversed array=w54:u8[])
            n194 = Type Cast(x=w64) -> (*(type *) &x=w63:string)  [unwired: 1 in]
            n195 = Split 1D Array(array=w54, index=w53) -> (first subarray=w51:u8[], second subarray=w52:u8[])
            n196 = Type Cast(type=w50, x=w52) -> (*(type *) &x=w65:u16)
            n197 = Coerce To Type(0:w65, 1:w66) -> (2:w48:T12)
            n198 = case shown="Default" w48 {
              tunnel: w59 -> [w80]
              frame Default {
                n199 = Get Date/Time In Seconds() -> (seconds since 1Jan1904=→"rx_packet ts":timestamp)
                "rx_packet" <- w80
              }
            }
            n200 = Type Cast(type=w50, x=w51) -> (*(type *) &x=w49:u16)
            n201 = case shown="\"Get Total State\"" w48 {
              tunnel: w64 -> [_ _ w108 _ _ _ _]
              tunnel: w63 -> [_ _ _ w113 w121 w129 w175]
              frame Default {
              }
              frame "None" {
              }
              frame "Get Total State" {
                w97 = dbl[] []  # double
                w103 = i32[] []  # i32
                w105 = 8  # 인덱스
                n202 = flat-sequence {
                  frame #0 {
                    n203 = Tick Count (ms)() -> (millisecond timer value=w110:u32)
                    n204 = feedback #4(w110) -> (w111:u32)
                    n205 = Subtract(x=w110, y=w111) -> (x-y=→"Get Total(Recv ms)":u32)
                    n206 = feedback-in #4(w110) -> ()
                  }
                }
                n207 = Reverse 1D Array(array=w108) -> (reversed array=w107:u8[])
                n208 = Split 1D Array(array=w107, index=w105) -> (first subarray=w102:u8[], second subarray=w106:u8[])
                n209 = Reverse 1D Array(array=w102) -> (reversed array=w101:u8[])
                n210 = Reverse 1D Array(array=w106) -> (reversed array=w96:u8[])
                n211 = Type Cast(x=w101) -> (*(type *) &x=w100:string)  [unwired: 1 in]
                n212 = Type Cast(x=w96) -> (*(type *) &x=w95:string)  [unwired: 1 in]
                n213 = call "reverseEndian32bit.vi"("In"=w100) -> ("Out"=w104:string)  [unwired: 9 in, 1 out]
                n214 = call "reverseEndian64bit.vi"("In"=w95) -> ("Out"=w98:string)  [unwired: 9 in, 1 out]
                n215 = Type Cast(type=w103, x=w104) -> (*(type *) &x=w99:i32[])
                n216 = Type Cast(type=w97, x=w98) -> (*(type *) &x=w94:dbl[])
                n217 = Index Array(array=w94) -> (element #1=w93:dbl, element #2=w92:dbl, element #3=w91:dbl, element #4=w90:dbl, element #5=w89:dbl, element #6=w88:dbl, element #7=w87:dbl)  [unwired: 7 in]
                n218 = Index Array(array=w99) -> (element #1=w86:i32, element #2=w82:i32)  [unwired: 2 in]
                n219 = Bundle(w86, w82) -> (w84:cluster{i32, i32})  [unwired: 1 in]
                n220 = Bundle(w93, w92, w91, w90) -> (w81:cluster{dbl, dbl, dbl, dbl})  [unwired: 1 in]
                n221 = Bundle(w89, w88, w87) -> (w85:cluster{dbl, dbl, dbl})  [unwired: 1 in]
                n222 = Bundle(w81, w85, w84) -> (→"Total State":T24)  [unwired: 1 in]
              }
              frame "Get Platform State" {
                w115 = i32[] []  # i32
                n223 = call "reverseEndian32bit.vi"("In"=w113) -> ("Out"=w114:string)  [unwired: 9 in, 1 out]
                n224 = Type Cast(type=w115, x=w114) -> (*(type *) &x=w116:i32[])
                n225 = flat-sequence {
                  frame #0 {
                    n226 = Tick Count (ms)() -> (millisecond timer value=w118:u32)
                    n227 = feedback #5(w118) -> (w119:u32)
                    n228 = Subtract(x=w118, y=w119) -> (x-y=→"Get Platform(Recv ms)":u32)
                    n229 = feedback-in #5(w118) -> ()
                  }
                }
                n230 = Array To Cluster(array=w116) -> (cluster=→"Platform State":cluster{"i32[0]":i32, "i32[1]":i32})
              }
              frame "Get Sensor State" {
                w122 = dbl[] []  # double
                n231 = call "reverseEndian64bit.vi"("In"=w121) -> ("Out"=w124:string)  [unwired: 9 in, 1 out]
                n232 = Type Cast(type=w122, x=w124) -> (*(type *) &x=w123:dbl[])
                n233 = flat-sequence {
                  frame #0 {
                    n234 = Tick Count (ms)() -> (millisecond timer value=w126:u32)
                    n235 = feedback #6(w126) -> (w127:u32)
                    n236 = Subtract(x=w126, y=w127) -> (x-y=→"Get Sensor(Recv ms)":u32)
                    n237 = feedback-in #6(w126) -> ()
                  }
                }
                n238 = Array To Cluster(array=w123) -> (cluster=→"Sensor State":T25)
              }
              frame "Get Position State" {
                w130 = dbl[] []  # double
                n239 = call "reverseEndian64bit.vi"("In"=w129) -> ("Out"=w132:string)  [unwired: 9 in, 1 out]
                n240 = Type Cast(type=w130, x=w132) -> (*(type *) &x=w131:dbl[])
                n241 = flat-sequence {
                  frame #0 {
                    n242 = Tick Count (ms)() -> (millisecond timer value=w134:u32)
                    n243 = feedback #7(w134) -> (w135:u32)
                    n244 = Subtract(x=w134, y=w135) -> (x-y=→"Get Position(Recv ms)":u32)
                    n245 = feedback-in #7(w134) -> ()
                  }
                }
                n246 = Array To Cluster(array=w131) -> (cluster=→"Position State":T26)
              }
              frame "Get Whisper State" {
                w141 = "%H:%M:%S%3u"  # format
                w164 = 11  # feed_pos
                w165 = 8  # cmd_pos
                w166 = 5  # vel
                w170 = 10  # index
                w171 = T11 {"subject"="", "value"=0.0}  # CustomValue
                n247 = flat-sequence {
                  frame #0 {
                    n248 = Tick Count (ms)() -> (millisecond timer value=w184:u32)
                    n249 = feedback #8(w184) -> (w185:u32)
                    n250 = Subtract(x=w184, y=w185) -> (x-y=→"Get Total(Recv ms)":u32)
                    n251 = feedback-in #8(w184) -> ()
                  }
                }
                n252 = call "reverseEndian64bit.vi"("In"=w175) -> ("Out"=w173:string)  [unwired: 9 in, 1 out]
                n253 = Format Date/Time String(time format string (%c)=w141) -> (date/time string=w140:string)  [unwired: 2 in]
                n254 = local read "saving?"() -> (w136:bool)
                n255 = Type Cast(type=T19 [], x=w173) -> (*(type *) &x=w172:T19)
                n256 = for {
                  tunnel: w172 -> [w196] mode=indexing
                  tunnel: w171 -> [w195]
                  tunnel: [w194] -> w167 mode=indexing
                  n257 = Unbundle(w196) -> ("subject"=w193:u64, "subject"=w187:i64, "val_dbl"=w191:dbl)
                  n258 = Type Cast(x=w187) -> (*(type *) &x=w189:string)  [unwired: 1 in]
                  n259 = Type Cast(x=w193) -> (*(type *) &x=w192:string)  [unwired: 1 in]
                  n260 = Reverse String(1:w189) -> (0:w188:string)
                  n261 = Reverse String(1:w192) -> (0:w190:string)
                  n262 = Concatenate Strings(w190, w188) -> (w186:string)
                  n263 = Bundle(cluster=w195, "subject"=w186, "value"=w191) -> (w194:T11)
                }
                n264 = Index Array(array=w167, index #1=w166, index #4=w165, index #7=w164) -> (element #1=w163:T11, element #2=w162:T11, element #3=w161:T11, element #4=w160:T11, element #5=w159:T11, element #6=w158:T11, element #7=w157:T11, element #8=w156:T11, element #9=w155:T11)  [unwired: 6 in]
                n265 = Split 1D Array(array=w167, index=w170) -> (first subarray=→"Whisper 1":T11[], second subarray=→"Whisper 2":T11[])
                n266 = Build Array(w163, w162, w161, w160, w159, w158, w157, w156, w155) -> (w154:T11[])
                n267 = for {
                  tunnel: w154 -> [w182] mode=indexing
                  tunnel: [w181] -> w142 mode=indexing
                  n268 = Unbundle(w182) -> ("value"=w181:dbl)  [unwired: 1 out]
                }
                n269 = for {
                  tunnel: w142 -> [w180] mode=indexing
                  tunnel: [w178] -> w139 mode=indexing
                  w179 = "%#.10f"  # format string
                  n270 = Format Value(format string=w179, value (0)=w180) -> (output string=w178:string)  [unwired: 1 in]
                }
                n271 = Build Array (concatenate)(w140, w139) -> (w138:string[])
                n272 = Build Array(w138) -> (w137:string[][])
                n273 = case shown="True" w136 {
                  tunnel: w137 -> [_ w176]
                  frame False {
                  }
                  frame True {
                    w177 = enumFgvFunction."Write"  # Function
                    n274 = call "saveData.vi"("body"=w176, "Function"=w177) -> ()  [unwired: 7 in, 3 out]
                  }
                }
                n275 = Index Array(array=w142) -> (element #1=w153:dbl, element #2=w152:dbl, element #3=w151:dbl, element #4=w150:dbl, element #5=w149:dbl, element #6=w148:dbl, element #7=w147:dbl, element #8=w146:dbl, element #9=w145:dbl)  [unwired: 9 in]
                n276 = Bundle("value"=w153, "value"=w152, "value"=w151) -> (→"vel 3" →"vel 4":cluster{"value":dbl, "value":dbl, "value":dbl})  [unwired: 1 in]
                n277 = Bundle("value"=w150, "value"=w149, "value"=w148, "value"=w147, "value"=w146, "value"=w145) -> (→"pos 3" →"pos 4":T9)  [unwired: 1 in]
              }
            }
            n278 = Get Date/Time In Seconds() -> (seconds since 1Jan1904=w47:timestamp)
            n279 = case shown="1" w49 {
              tunnel: w48 -> [_ w72 w74 w76 w78]
              tunnel: w47 -> [_ w71 w73 w75 w77]
              frame Default {
              }
              frame 1 {
                "ACK ts" <- w71
                "ACK Command" <- w72
              }
              frame 2 {
                "RES ts" <- w73
                "RES Command" <- w74
              }
              frame 4 {
                "ONE" <- w75
                "ONE Command" <- w76
              }
              frame 8 {
                "STREAM" <- w77
                "STREAM Command" <- w78
              }
            }
          }
        }
        n280 = local read "stop"() -> (w45:bool)
      }
      n281 = Merge Errors(w31, w34, w29) -> (w33:errorcluster)
    }
    frame Error {
      w421 = "ROS Master is not response!!"  # message
      n282 = One Button Dialog(message=w421) -> ()  [unwired: 1 in, 1 out]
    }
  }
  n283 = flat-sequence {
    tunnel: w2 -> [_]
    frame #0 {
      w424 = T16."Run Time System"  # Application:Kind
      n284 = property class="App"() -> ("App.Kind"=w425:T16)  [unwired: 2 in, 2 out]
      n285 = Equal?(x=w425, y=w424) -> (x = y?=w423:bool)
      n286 = case shown="True" w423 {
        selector: w423 -> [_ w426]
        frame False {
        }
        frame True {
          n287 = flat-sequence {
            tunnel: w426 -> [w427]
            frame #0 {
              n288 = invoke class="VI" method="FP.Close"() -> ()  [unwired: 3 in, 3 out]
            }
            frame #1 {
              n289 = Quit LabVIEW(quit? (T)=w427) -> ()
            }
          }
        }
      }
    }
  }
